vi "2020.vi"() -> ()   [LabVIEW 2025]
doc: "撒旦发生发生"
panel:
  out "Slide 4":u8(slide) scale=0.0..100.0
  in  "Slide 3":dbl(slide) scale=0.0..10.0
  in  "Slide 2":dbl(slide) scale=0.0..10.0
  in  "Slide":dbl(slide) scale=0.0..10.0
  in  "Numeric":dbl
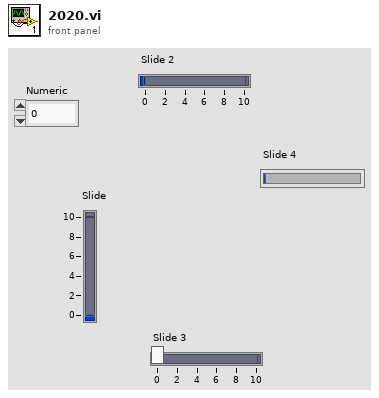
[diagram p1: front panel]
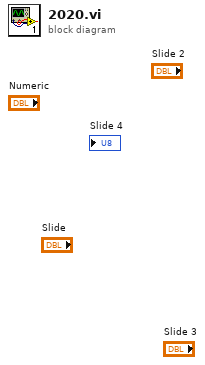
[diagram p0: block diagram]
diagram:
